vi "ClusterwithUNDEFINEDTYPE.vi"(1 "Cluster In":cluster{}) -> (0 "Cluster Out":cluster{})   [LabVIEW 2010]
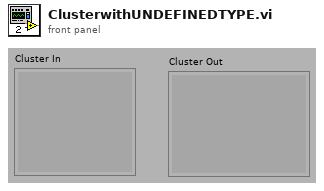
[diagram p1: front panel]
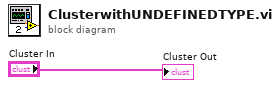
[diagram p0: block diagram]
diagram:
  "Cluster Out" <- "Cluster In"
